vi "Get Supported Music File Paths.vi"(8 "error in (no error)":errorcluster, 10 "Music Folder Path":path, 11 "MusicFile In":refnum<class "MusicFile.lvclass">) -> (0 "error out":errorcluster, 2 "Music File Paths":path[](array[path]), 3 "MusicFile Out":refnum<class "MusicFile.lvclass">)   [LabVIEW 2015, in "MusicFile.lvclass"]
uses:
  MusicFile.lvclass
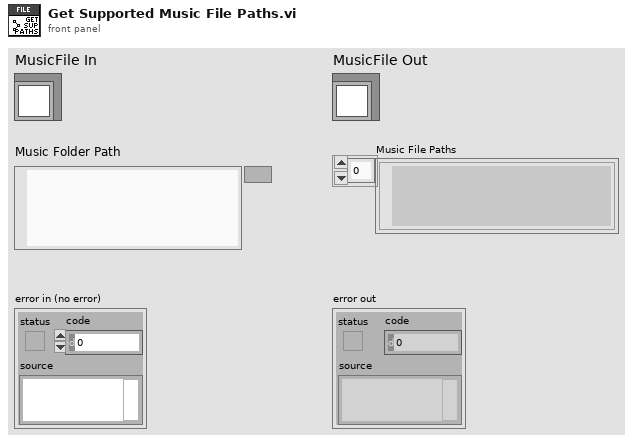
[diagram p1: front panel]
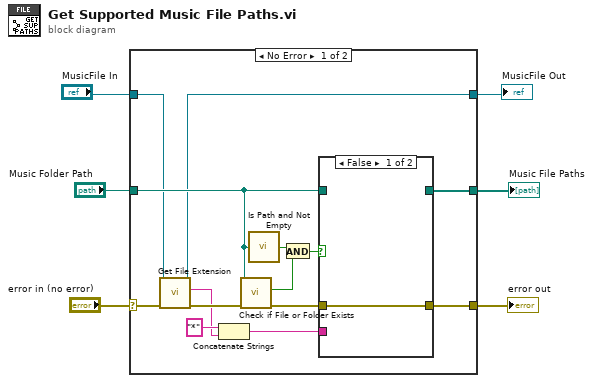
[diagram p0: block diagram]
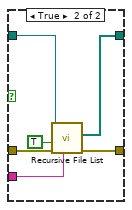
[diagram p2: hidden frame]
diagram:
  n1 = case shown="No Error" "error in (no error)" {
    selector: "error in (no error)" -> [w11 w29]
    tunnel: [w18 w29] -> w5
    tunnel: [w8 w28] -> w1
    tunnel: "MusicFile In" -> [w9 w28]
    tunnel: "Music Folder Path" -> [w15 _]
    tunnel: [w17 _] -> w3
    frame No Error {
      n2 = call-dynamic "Get File Extension.vi"("error in (no error)"=w11, "MusicFile"=w9) -> ("error out"=w10:errorcluster, "File Extention"=w7:string, "MusicFile"=w8:refnum<class "MusicFile.lvclass">)  [unwired: 7 in]
      n3 = Concatenate Strings("*" ("string"), w7) -> (w19:string)
      n4 = call <vilib>:"Check if File or Folder Exists.vi"("error in (no error)"=w10, "path"=w15) -> ("error out"=w16:errorcluster, "file or folder exists?"=w13:bool)  [unwired: 7 in, 1 out]
      n5 = call <vilib>:"Is Path and Not Empty.vi"("path"=w15) -> ("Is Path and Not Empty?"=w14:bool)  [unwired: 4 in]
      n6 = And(x=w14, y=w13) -> (x .and. y?=w12:bool)
      n7 = case shown="False" w12 {
        tunnel: w19 -> [_ w26]
        tunnel: [w21 w25] -> w18
        tunnel: [_ w24] -> w17
        tunnel: w15 -> [_ w23]
        tunnel: w16 -> [w21 w22]
        frame False {
        }
        frame True {
          n8 = call <vilib>:"Recursive File List.vi"("pattern"=w26, "error in (no error)"=w22, "Continue Recursing on Error? (F)"=TRUE, "Folder Path"=w23) -> ("error out"=w25:errorcluster, "All Files in Dir"=w24:path[])  [unwired: 3 in, 3 out]
        }
      }
    }
    frame Error {
    }
  }
  "error out" <- w5
  "Music File Paths" <- w3
  "MusicFile Out" <- w1
